vi "Get HardwareUUID.vi"(8 "error in (no error)":errorcluster, 11 "Output Actor Hardware in":refnum<class "Output Actor Hardware.lvclass">) -> (0 "error out":errorcluster, 2 "UUID":string, 3 "Output Actor Hardware out":refnum<class "Output Actor Hardware.lvclass">)   [LabVIEW 2015, in "Output Actor Hardware.lvclass"]
uses:
  Output Actor Hardware.lvclass
  Output Actor Hardware.lvclass/Output Actor Hardware.ctl
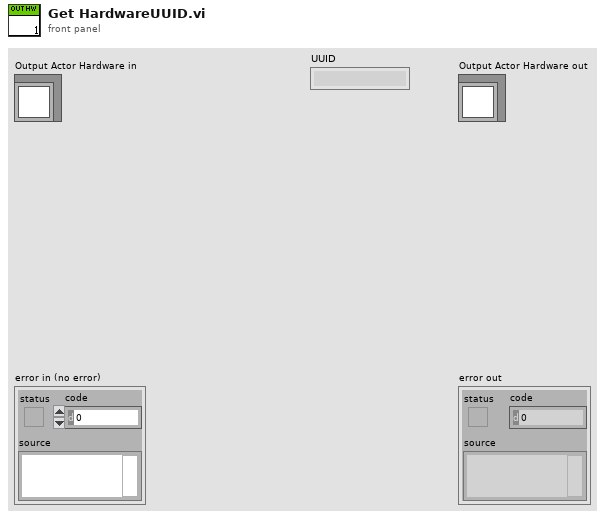
[diagram p1: front panel]
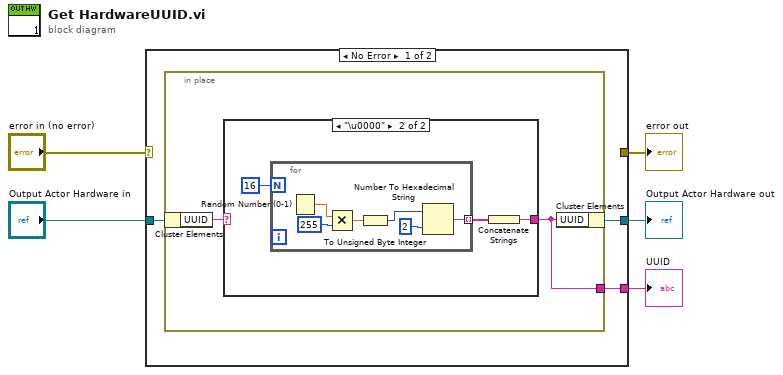
[diagram p0: block diagram]
diagram:
  n1 = case shown="No Error" "error in (no error)" {
    selector: "error in (no error)" -> [_ w22]
    tunnel: [_ w22] -> w4
    tunnel: [w6 w21] -> w2
    tunnel: "Output Actor Hardware in" -> [w8 w21]
    tunnel: [w7 _] -> w1
    frame No Error {
      n2 = in-place {
        in-place-border: [w9] -> w7
        n3 = in-place-cluster #1(w8) -> ("UUID"=w10:string)
        n4 = case shown="\"\"" w10 {
          selector: w10 -> [w11 _]
          tunnel: [w11 w12] -> w9
          frame "False", Default {
          }
          frame "\u0000" {
            n5 = for {
              N: 16 -> [_]
              tunnel: [w15] -> w14 mode=indexing
              n6 = Random Number (0-1)() -> (number: 0 to 1=w20:dbl)
              n7 = Multiply(x=w20, y=255) -> (x*y=w18:dbl)
              n8 = To Unsigned Byte Integer(number=w18) -> (unsigned 8bit integer=w17:u8)
              n9 = Number To Hexadecimal String(1:i16 2 ("width (-)"), 2:w17) -> (0:w15:string)
            }
            n10 = Concatenate Strings(w14) -> (w12:string)
          }
        }
        n11 = in-place-cluster #1("UUID"=w9) -> (w6:refnum<class "Output Actor Hardware.lvclass">)
      }
    }
    frame Error {
    }
  }
  "error out" <- w4
  "Output Actor Hardware out" <- w2
  "UUID" <- w1
